vi "Realtime_interaction VI.vi"() -> ()   [LabVIEW 2020]
uses:
  <vilib>/rvi/interface/nirviOpenFPGA/nirviOpenFPGA.xnode
  <vilib>/rvi/interface/nirviReadWriteControl/nirviReadWriteControl.xnode
  <vilib>/rvi/interface/nirviCloseFPGA/nirviCloseFPGA.xnode
  <vilib>/FPGAPlugInAG/Dynamic/niLvFpga_Close_Dynamic.vi
  NiFpgaLv.dll
  <vilib>/Utility/error.llb/Error Cluster From Error Code.vi
  <vilib>/rvi/interface/Simulation/niFpgaSimulationCallBeginRW.vi
  <vilib>/rvi/errors/niLvFpgaAdjustHostInterfaceError.vi
  New folder/FPGA_controlled VI.vi
  <vilib>/FPGAPlugInAG/cRIO-9054/niLvFpga_Open_cRIO-9054.vi
  <vilib>/rvi/interface/common/dynamic/niFpgaDynamicAddResources.vi
  FPGA Bitfiles/ver0.1_FPGATarget_FPGAcontrolledVI_cWk4O34ijhk.lvbitx
panel:
  out "Boolean":bool
  out "millisecond timer value":u32
  out "Mod1/AI0":fxp<+/-,26,5>
  in  "stop":bool
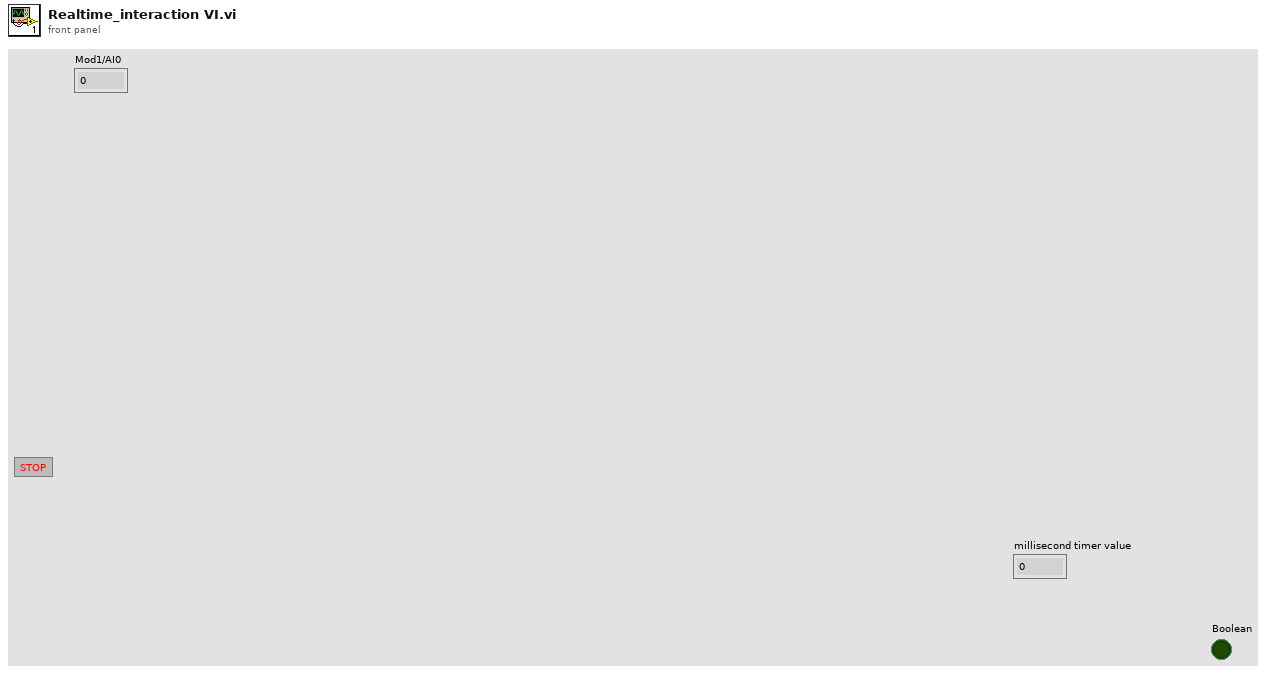
[diagram p1: front panel]
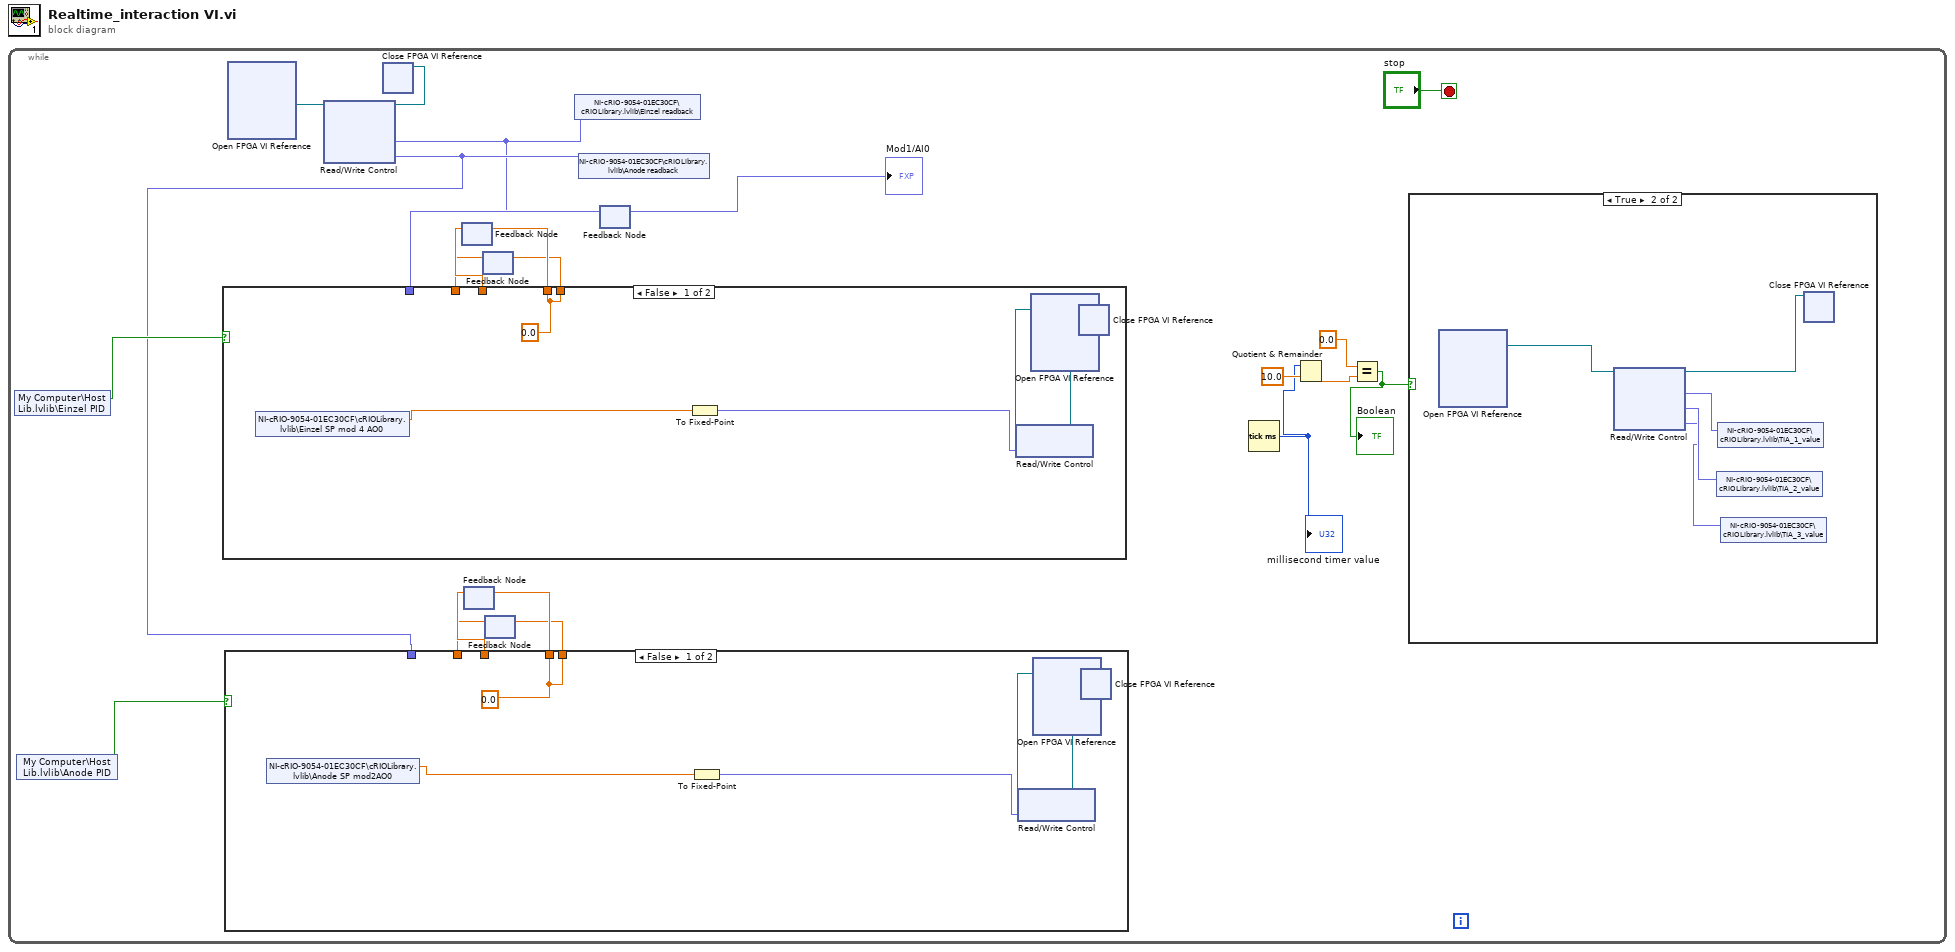
[diagram p0: block diagram]
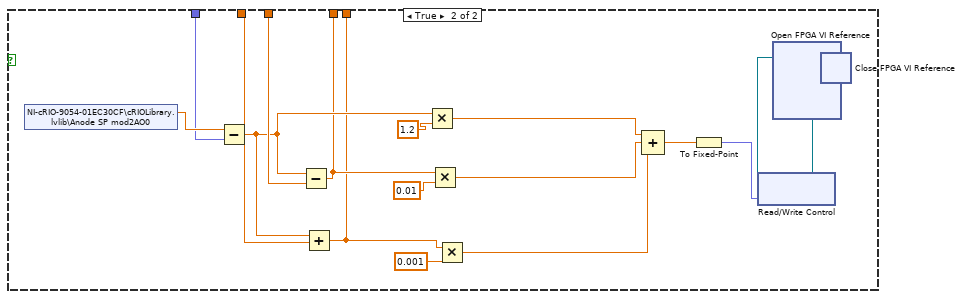
[diagram p3: hidden frame]
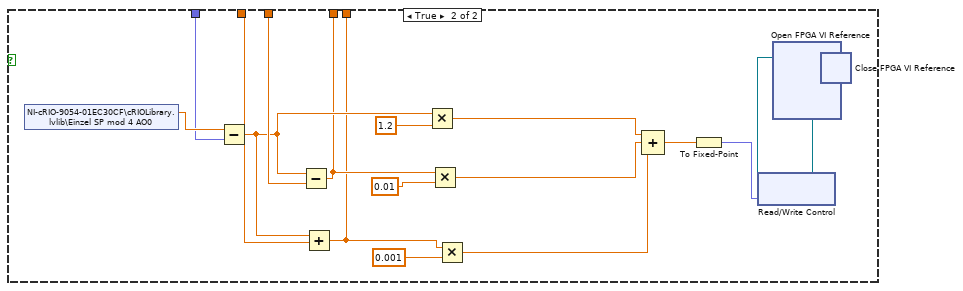
[diagram p4: hidden frame]
diagram:
  n1 = while {
    stop <- "stop" stop-if-true
    n2 = shared-variable "My Computer\\Host Lib.lvlib\\Einzel PID"() -> (w18:bool)  [unwired: 1 in, 1 out]
    n3 = shared-variable "My Computer\\Host Lib.lvlib\\Anode PID"() -> (w12:bool)  [unwired: 1 in, 1 out]
    n4 = xnode "Open FPGA VI Reference"() -> ("FPGA VI Reference Out"=w20:refnum<k20>)  [unwired: 2 in, 1 out]
    n5 = xnode "Read/Write Control"("FPGA VI Reference In"=w20) -> ("FPGA VI Reference Out"=w19:refnum<k20>, "Mod1/AI0"=w6:fxp<+/-,26,5>, "Mod1/AI2"=w7:fxp<+/-,26,5>)  [unwired: 2 in, 1 out]
    n6 = xnode "Close FPGA VI Reference"("FPGA VI Reference In"=w19) -> ()  [unwired: 1 in, 1 out]
    n7 = feedback #1() -> (w15:dbl)  [unwired: 1 in]
    n8 = feedback #2() -> (w10:dbl)  [unwired: 1 in]
    n9 = feedback #3() -> (w13:dbl)  [unwired: 1 in]
    n10 = feedback #4() -> (w8:dbl)  [unwired: 1 in]
    n11 = case shown="False" w12 {
      tunnel: w7 -> [_ w47]
      tunnel: w10 -> [_ w46]
      tunnel: [w27 w43] -> w11
      tunnel: [w27 w41] -> w9
      tunnel: w8 -> [_ w44]
      frame False {
        w27 = 0.0
        n12 = shared-variable "NI-cRIO-9054-01EC30CF\\cRIOLibrary.lvlib\\Anode SP mod2AO0"() -> (w28:dbl)  [unwired: 1 in, 1 out]
        n13 = To Fixed-Point(number=w28) -> (fixed-point=w29:fxp<+/-,20,5>)  [unwired: 1 in]
        n14 = xnode "Open FPGA VI Reference"() -> ("FPGA VI Reference Out"=w30:refnum<k20>)  [unwired: 2 in, 1 out]
        n15 = xnode "Read/Write Control"("FPGA VI Reference In"=w30, "Mod2/AO0"=w29) -> ("FPGA VI Reference Out"=w31:refnum<k20>)  [unwired: 1 in, 1 out]
        n16 = xnode "Close FPGA VI Reference"("FPGA VI Reference In"=w31) -> ()  [unwired: 1 in, 1 out]
      }
      frame True {
        n17 = shared-variable "NI-cRIO-9054-01EC30CF\\cRIOLibrary.lvlib\\Anode SP mod2AO0"() -> (w48:dbl)  [unwired: 1 in, 1 out]
        n18 = Subtract(x=w48, y=w47) -> (x-y=w45:dbl)
        n19 = Subtract(x=w45, y=w46) -> (x-y=w43:dbl)
        n20 = Add(x=w45, y=w44) -> (x+y=w41:dbl)
        n21 = Multiply(x=w45, y=1.2) -> (x*y=w40:dbl)
        n22 = Multiply(x=w43, y=0.01) -> (x*y=w42:dbl)
        n23 = Multiply(x=w41, y=0.001) -> (x*y=w39:dbl)
        n24 = Compound Arithmetic op=ADD(w40, w42, w39) -> (w35:dbl)
        n25 = To Fixed-Point(number=w35) -> (fixed-point=w36:fxp<+/-,20,5>)  [unwired: 1 in]
        n26 = xnode "Open FPGA VI Reference"() -> ("FPGA VI Reference Out"=w38:refnum<k20>)  [unwired: 2 in, 1 out]
        n27 = xnode "Read/Write Control"("FPGA VI Reference In"=w38, "Mod2/AO0"=w36) -> ("FPGA VI Reference Out"=w37:refnum<k20>)  [unwired: 1 in, 1 out]
        n28 = xnode "Close FPGA VI Reference"("FPGA VI Reference In"=w37) -> ()  [unwired: 1 in, 1 out]
      }
    }
    n29 = feedback-in #2(w11) -> ()
    n30 = feedback-in #4(w9) -> ()
    n31 = shared-variable "NI-cRIO-9054-01EC30CF\\cRIOLibrary.lvlib\\Einzel readback"(w6) -> ()  [unwired: 1 in, 1 out]
    n32 = shared-variable "NI-cRIO-9054-01EC30CF\\cRIOLibrary.lvlib\\Anode readback"(w7) -> ()  [unwired: 1 in, 1 out]
    n33 = feedback-in #5(w6) -> ()
    n34 = feedback #5() -> (w17:fxp<+/-,26,5>)  [unwired: 1 in]
    "Mod1/AI0" <- w17
    n35 = case shown="False" w18 {
      tunnel: w17 -> [_ w69]
      tunnel: w15 -> [_ w68]
      tunnel: [w50 w65] -> w16
      tunnel: [w50 w63] -> w14
      tunnel: w13 -> [_ w66]
      frame False {
        w50 = 0.0
        n36 = shared-variable "NI-cRIO-9054-01EC30CF\\cRIOLibrary.lvlib\\Einzel SP mod 4 AO0"() -> (w49:dbl)  [unwired: 1 in, 1 out]
        n37 = To Fixed-Point(number=w49) -> (fixed-point=w51:fxp<+/-,20,5>)  [unwired: 1 in]
        n38 = xnode "Open FPGA VI Reference"() -> ("FPGA VI Reference Out"=w52:refnum<k20>)  [unwired: 2 in, 1 out]
        n39 = xnode "Read/Write Control"("FPGA VI Reference In"=w52, "Mod4/AO0"=w51) -> ("FPGA VI Reference Out"=w53:refnum<k20>)  [unwired: 1 in, 1 out]
        n40 = xnode "Close FPGA VI Reference"("FPGA VI Reference In"=w53) -> ()  [unwired: 1 in, 1 out]
      }
      frame True {
        n41 = shared-variable "NI-cRIO-9054-01EC30CF\\cRIOLibrary.lvlib\\Einzel SP mod 4 AO0"() -> (w70:dbl)  [unwired: 1 in, 1 out]
        n42 = Subtract(x=w70, y=w69) -> (x-y=w67:dbl)
        n43 = Subtract(x=w67, y=w68) -> (x-y=w65:dbl)
        n44 = Add(x=w67, y=w66) -> (x+y=w63:dbl)
        n45 = Multiply(x=w67, y=1.2) -> (x*y=w62:dbl)
        n46 = Multiply(x=w65, y=0.01) -> (x*y=w64:dbl)
        n47 = Multiply(x=w63, y=0.001) -> (x*y=w61:dbl)
        n48 = Compound Arithmetic op=ADD(w62, w64, w61) -> (w57:dbl)
        n49 = To Fixed-Point(number=w57) -> (fixed-point=w58:fxp<+/-,20,5>)  [unwired: 1 in]
        n50 = xnode "Open FPGA VI Reference"() -> ("FPGA VI Reference Out"=w60:refnum<k20>)  [unwired: 2 in, 1 out]
        n51 = xnode "Read/Write Control"("FPGA VI Reference In"=w60, "Mod4/AO0"=w58) -> ("FPGA VI Reference Out"=w59:refnum<k20>)  [unwired: 1 in, 1 out]
        n52 = xnode "Close FPGA VI Reference"("FPGA VI Reference In"=w59) -> ()  [unwired: 1 in, 1 out]
      }
    }
    n53 = feedback-in #1(w16) -> ()
    n54 = feedback-in #3(w14) -> ()
    n55 = Tick Count (ms)() -> (millisecond timer value=w4:u32)
    "millisecond timer value" <- w4
    n56 = Quotient & Remainder(x=w4, y=10.0) -> (x-y*floor(x/y)=w3:dbl)  [unwired: 1 out]
    n57 = Equal?(x=0.0, y=w3) -> (x = y?=w1:bool)
    "Boolean" <- w1
    n58 = case shown="True" w1 {
      frame False {
      }
      frame True {
        n59 = xnode "Open FPGA VI Reference"() -> ("FPGA VI Reference Out"=w26:refnum<k20>)  [unwired: 2 in, 1 out]
        n60 = xnode "Read/Write Control"("FPGA VI Reference In"=w26) -> ("FPGA VI Reference Out"=w25:refnum<k20>, "Mod1/AI7"=w24:fxp<+/-,26,5>, "Mod1/AI8"=w23:fxp<+/-,26,5>, "Mod1/AI9"=w22:fxp<+/-,26,5>)  [unwired: 1 in, 1 out]
        n61 = shared-variable "NI-cRIO-9054-01EC30CF\\cRIOLibrary.lvlib\\TIA_2_value"(w23) -> ()  [unwired: 1 in, 1 out]
        n62 = shared-variable "NI-cRIO-9054-01EC30CF\\cRIOLibrary.lvlib\\TIA_1_value"(w24) -> ()  [unwired: 1 in, 1 out]
        n63 = shared-variable "NI-cRIO-9054-01EC30CF\\cRIOLibrary.lvlib\\TIA_3_value"(w22) -> ()  [unwired: 1 in, 1 out]
        n64 = xnode "Close FPGA VI Reference"("FPGA VI Reference In"=w25) -> ()  [unwired: 1 in, 1 out]
      }
    }
  }
